vi "build_linear_array type2.vi"(9 "begin":dbl=10.0, 10 "d":dbl=10.0, 11 "#":i32=10) -> (3 "1D Array output":dbl[](array[numeric]))   [LabVIEW 2011]
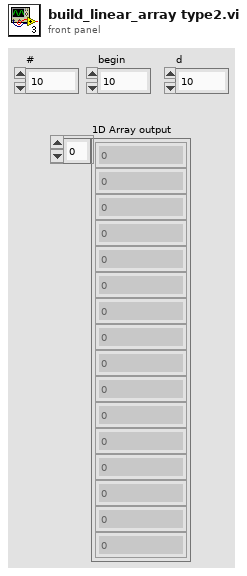
[diagram p1: front panel]
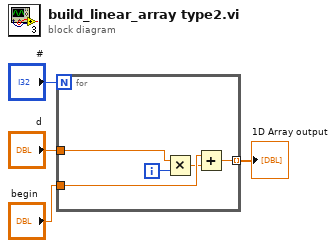
[diagram p0: block diagram]
diagram:
  n1 = for {
    N: "#" -> [_]
    tunnel: "d" -> [w5]
    tunnel: "begin" -> [w8]
    tunnel: [w6] -> w1 mode=indexing
    i -> [w9]
    n2 = Multiply(x=w5, y=w9) -> (x*y=w7:dbl)
    n3 = Add(x=w8, y=w7) -> (x+y=w6:dbl)
  }
  "1D Array output" <- w1
